vi "DeleteDependency.vi"(8 "error in (no error)":errorcluster, 9 "Item to depend on":refnum<class "ILabVIEWItem.lvclass">, 11 "CLabVIEWItem in":refnum<class "CLabVIEWItem.lvclass">) -> (0 "error out":errorcluster, 3 "CLabVIEWItem out":refnum<class "CLabVIEWItem.lvclass">)   [LabVIEW 2020, in "LabVIEWItem.lvlib" / "CLabVIEWItem.lvclass"]
uses:
  CLabVIEWItem.lvclass
  obj/Addons/LabVIEWObjectInterfaces.lvlibp/LabVIEWObjectInterfaces/ILabVIEWItem/ILabVIEWItem.lvclass
  CLabVIEWItem.lvclass/CLabVIEWItem.ctl
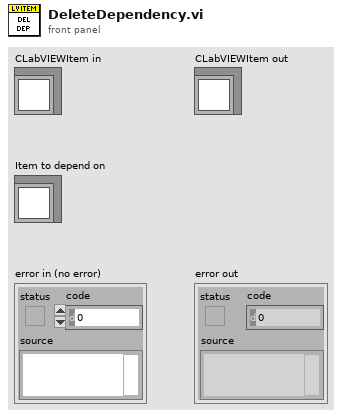
[diagram p1: front panel]
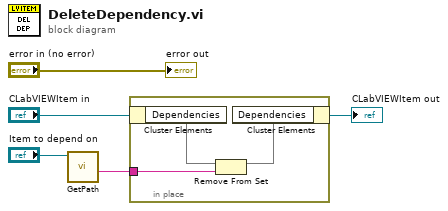
[diagram p0: block diagram]
diagram:
  n1 = call-dynamic "GetPath.vi"("ILabVIEWItem in"="Item to depend on") -> ("Path"=w2:string)  [unwired: 8 in, 2 out]
  n2 = in-place {
    in-place-border: w2 -> [w6]
    n3 = in-place-cluster #1("CLabVIEWItem in") -> ("Dependencies"=w8:set{string})
    n4 = Remove From Set(10:w6, 11:w8) -> (3:w7:set{string})  [unwired: 1 out]
    n5 = in-place-cluster #1("Dependencies"=w7) -> (→"CLabVIEWItem out":refnum<class "CLabVIEWItem.lvclass">)
  }
  "error out" <- "error in (no error)"
